vi "DB - Columns INFO.vi"(0 "Refnum in":T3, 1 "subVI (auto)":bool=TRUE, 5 "DB.dbo.Table":string="SRTRS.MasterData.Procedure", 11 "error in (no error)":errorcluster) -> (2 "IDENTITY COLUMN":string, 3 "Table Description":string, 4 "Refnum out":T3, 6 "COLUMN_NAME":string[](array[string]), 8 "DATA_TYPE":string[](array[string]), 10 "PRECISION":string[](array[string]), 13 "COUNT":i32, 14 "MS_Description":string[](array[string]), 15 "error out":errorcluster)   [LabVIEW 2013]
uses:
  <vilib>/addons/database/Connection.llb/Conn ObjectReference.ctl
  Controls/DB - DB.Schema.Table.ctl
  <vilib>/addons/database/Connection.llb/Conn Execute.vi
  <vilib>/addons/database/Recordset.llb/Rec Fetch String Data (R).vi
  <vilib>/addons/database/Recordset.llb/Rec Destroy - Connection.vi
  <vilib>/addons/database/Recordset.llb/Rec Fetch Recordset Data (R).vi
  <vilib>/addons/database/Connection.llb/DB Tools Open Connec (String).vi
  <vilib>/addons/database/_DB Variant To Data/Database Variant To Data.xnode
  <vilib>/addons/database/NI_Database_API.lvlib
panel:
  out "# of SQL Statements":i32
  out "Fetch = 0 Error":errorcluster
  out "isIdentity":string[](array[string])
  out "SQL Statement":string[](array[string])
  out "String":string
  out "DB.Schema.Table":T1
  out "call chain":string[](array[string])
  out "data":string[][](array[string])
  in  "Connection Information":T2={"Connection "="SQL Server 32bit HPEnvy", "Username"="admin", "Password"="admin123"}
  # "Orders\nPartsDetails\nTransactions"
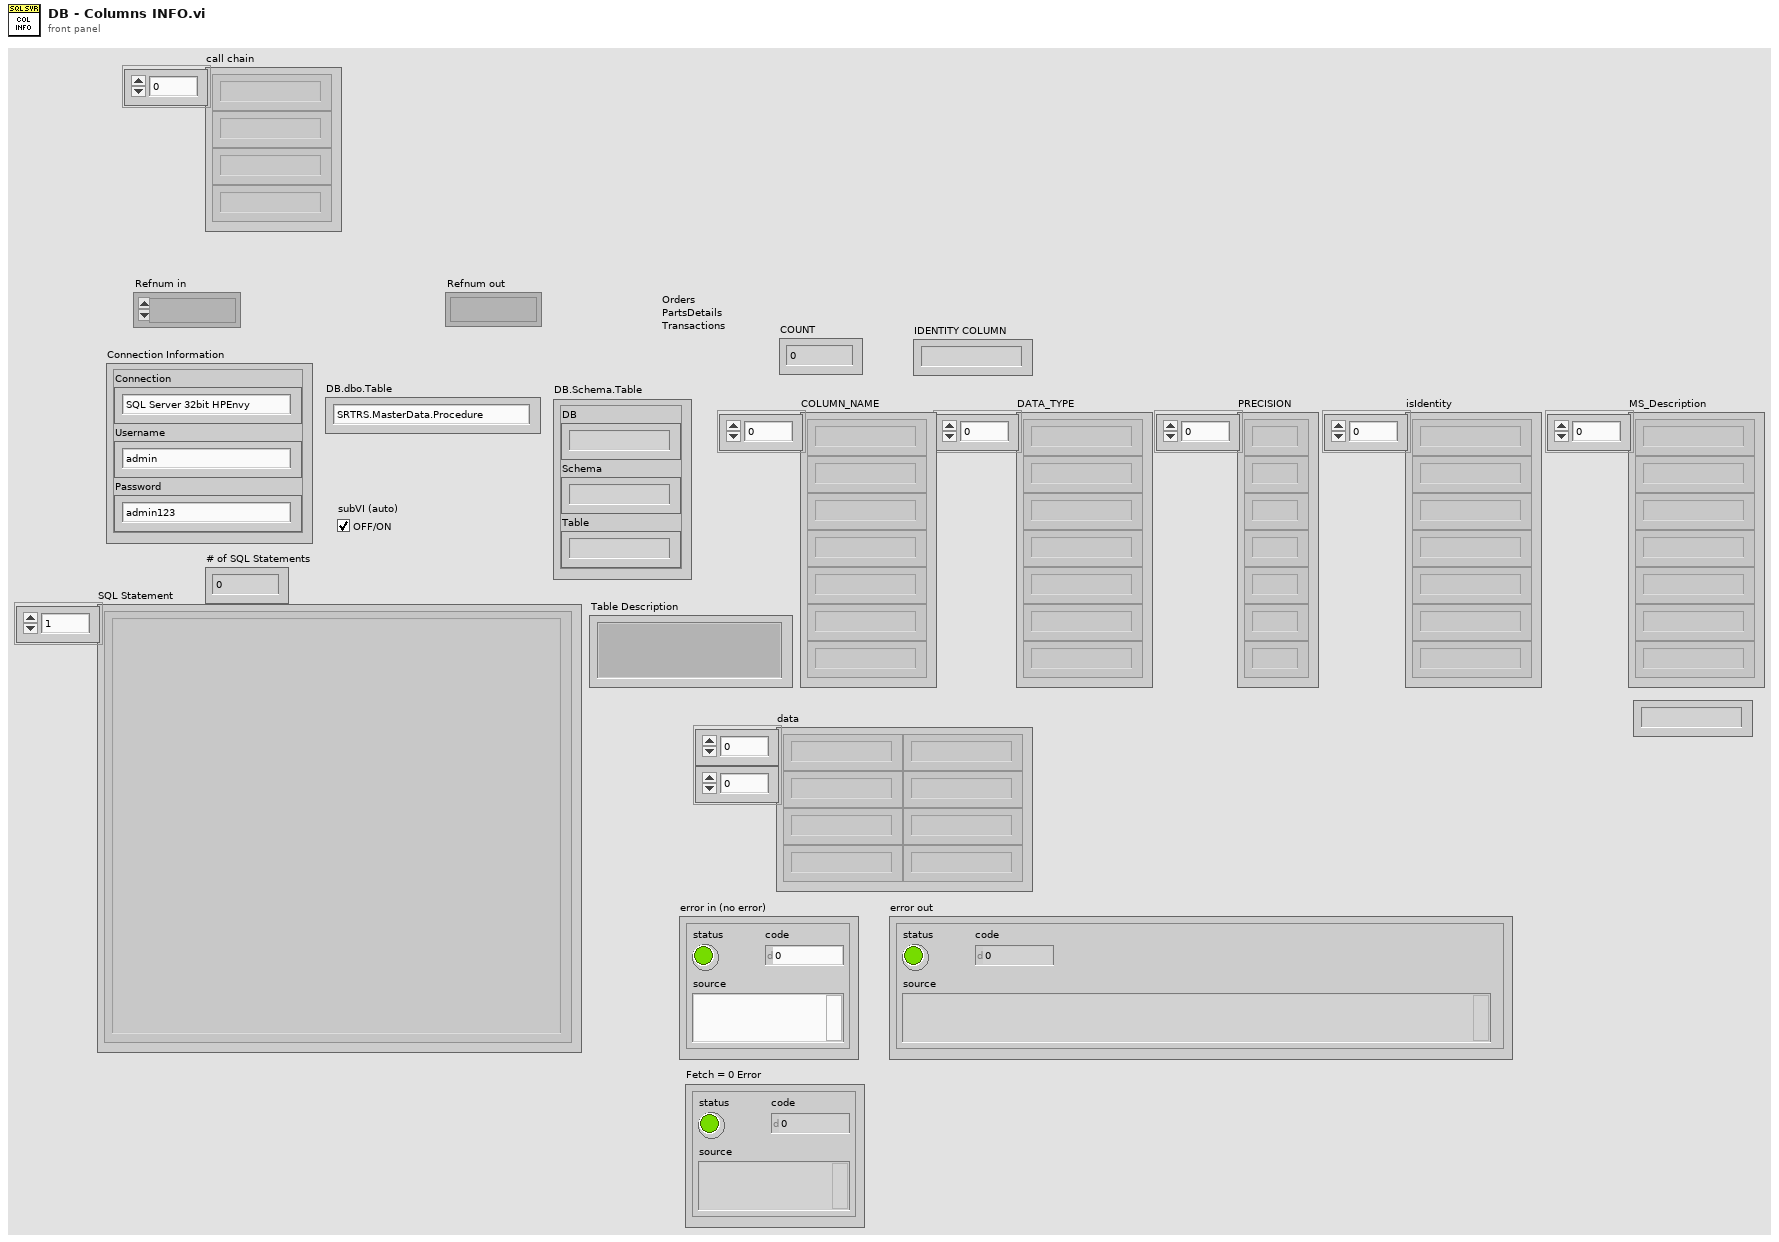
[diagram p1: front panel]
types:
  T1 = typedef "DB - DB.Schema.Table.ctl" = cluster{"DB":string, "Schema":string, "Table":string}
  T2 = cluster{"Connection ":string, "Username":string, "Password":string}
  T3 = typedef "NI_Database_API.lvlib/Conn ObjectReference.ctl" = refnum<k1>
  T4 = typedef "NI_Database_API.lvlib/Rec ObjectReference.ctl" = refnum<k1>
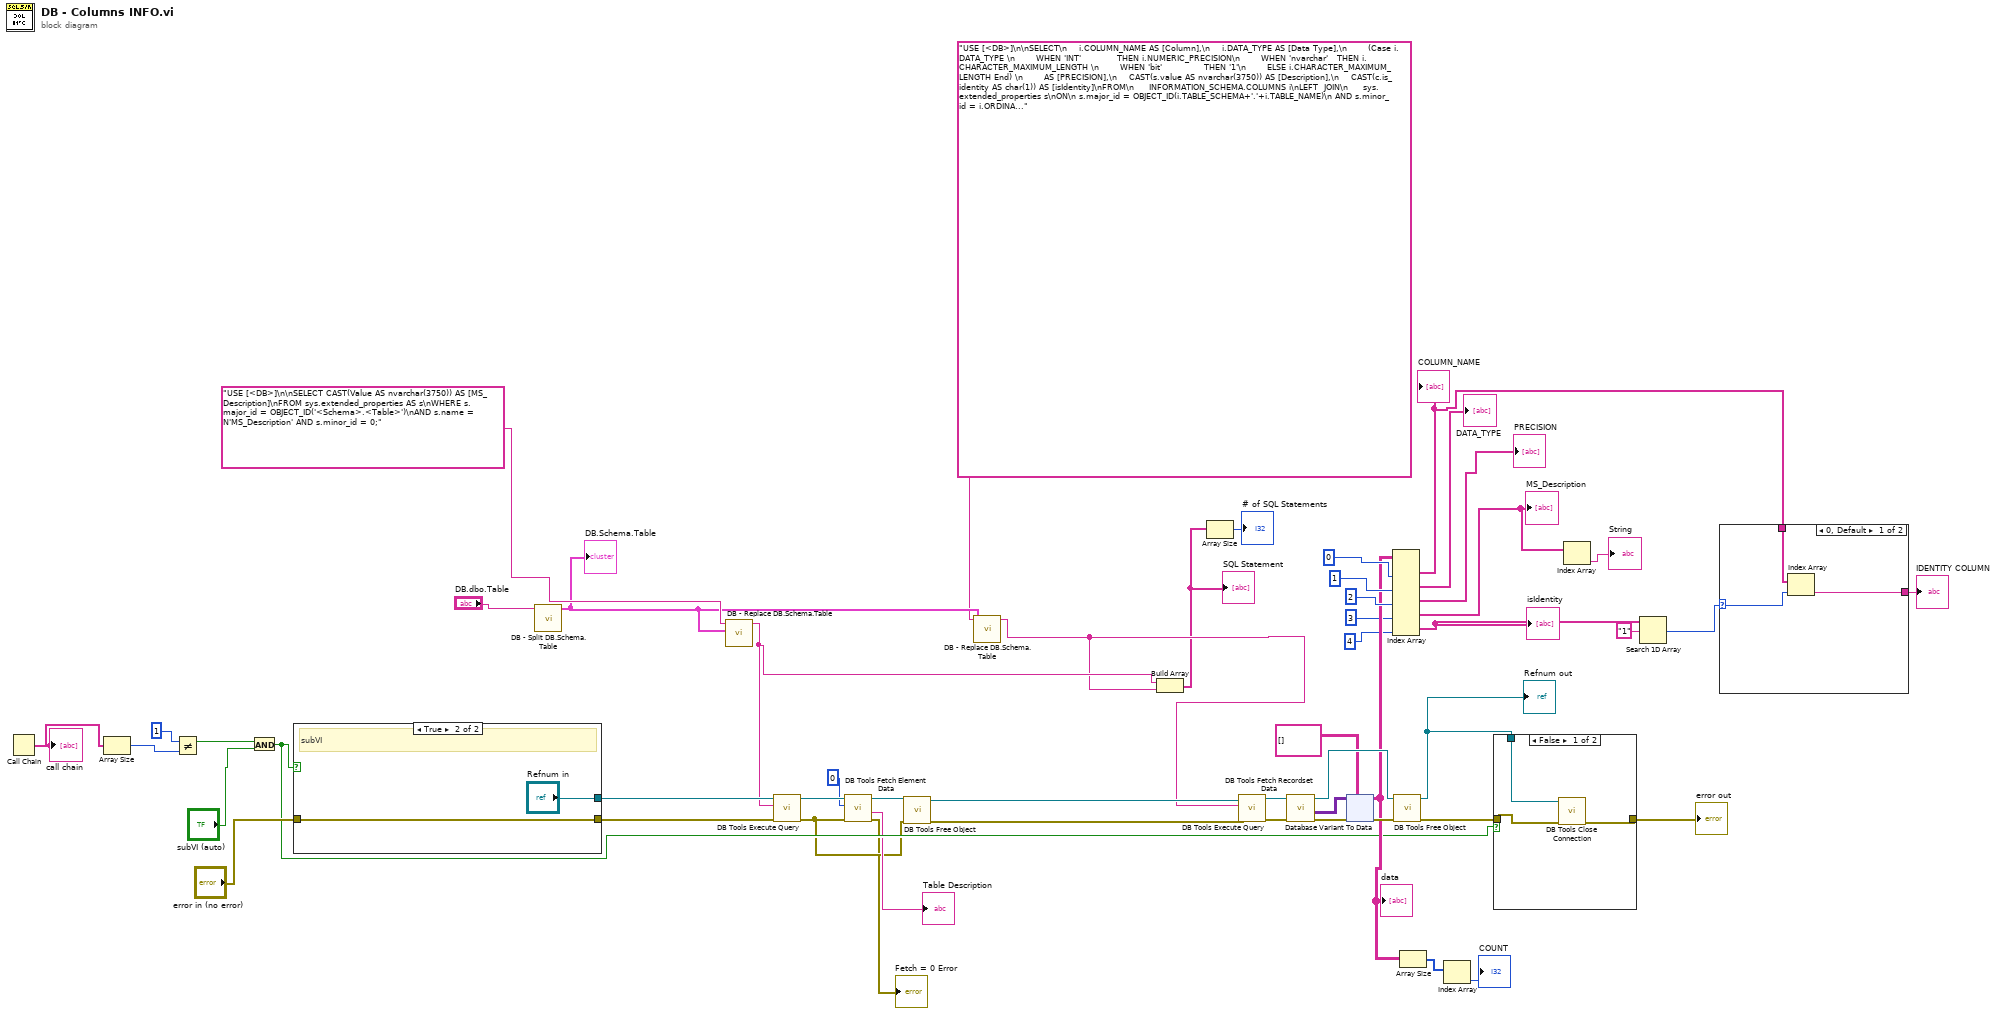
[diagram p0: block diagram]
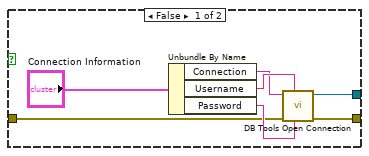
[diagram p4: hidden frame]
diagram:
  n1 = Call Chain() -> (call chain=w32:string[])
  "call chain" <- w32
  n2 = Array Size(array=w32) -> (size(s)=w31:i32)
  n3 = Not Equal?(x=1, y=w31) -> (x != y?=w30:bool)
  n4 = And(x=w30, y="subVI (auto)") -> (x .and. y?=w27:bool)
  n5 = case shown="True" w27 {
    tunnel: [w55 "Refnum in"] -> w21
    tunnel: "error in (no error)" -> [w54 w60]
    tunnel: [w53 w60] -> w20
    frame False {
      n6 = Unbundle By Name("Connection Information") -> ("Connection"=w57:string, "Username"=w58:string, "Password"=w56:string)
      n7 = call-poly <vilib>:"DB Tools Open Connection.vi"("password"=w56, "userID"=w58, "error in (no error)"=w54, "connection information"=w57) -> ("error out"=w53:errorcluster, "connection reference"=w55:T3)  [unwired: 4 in]
    }
    frame True {
      # "subVI"
    }
  }
  n8 = call "DB - Split DB.Schema.Table.vi"("DB.Schema.Table"="DB.dbo.Table") -> ("DB.Schema.Table"=w22:T1)  [unwired: 10 in]
  "DB.Schema.Table" <- w22
  n9 = call "DB - Replace DB.Schema.Table.vi"("DB.Schema.Table"=w22, "string in"="USE [<DB>]\n\nSELECT CAST(Value AS nvarchar(3750)) AS [MS_Description]\nFROM sys.extended_properties AS s\nWHERE s.major_id = OBJECT_ID('<Schema>.<Table>')\nAND s.name = N'MS_Description' AND s.minor_id = 0;") -> ("string out"=w16:string)  [unwired: 8 in, 1 out]
  n10 = call-poly <vilib>:"DB Tools Execute Query.vi"("error in (no error)"=w20, "SQL query"=w16, "connection reference"=w21) -> ("error out"=w4:errorcluster, "recordset reference"=w7:T4)  [unwired: 5 in]
  n11 = call-poly <vilib>:"DB Tools Fetch Element Data.vi"("error in (no error)"=w4, "column index"=0, "recordset reference"=w7) -> ("error out"=→"Fetch = 0 Error":errorcluster, "data"=→"Table Description":string, "recordset reference out"=w19:T4)  [unwired: 4 in]
  n12 = call-poly <vilib>:"DB Tools Free Object.vi"("error in (no error)"=w4, "recordset reference"=w19) -> ("error out"=w17:errorcluster, "connection reference"=w18:T3)  [unwired: 8 in]
  n13 = call "DB - Replace DB.Schema.Table.vi"("DB.Schema.Table"=w22, "string in"="USE [<DB>]\n\nSELECT\n    i.COLUMN_NAME AS [Column],\n    i.DATA_TYPE AS [Data Type],\n       (Case i.DATA_TYPE \n       WHEN 'INT'            THEN i.NUMERIC_PRECISION\n       WHEN 'nvarchar'   THEN i.CHARACTER_MAXIMUM_LENGTH \n       WHEN 'bit'              THEN '1'\n       ELSE i.CHARACTER_MAXIMUM_LENGTH End) \n       AS [PRECISION],\n    CAST(s.value AS nvarchar(3750)) AS [Description],\n    CAST(c.is_identity AS char(1)) AS [isIdentity]\nFROM\n     INFORMATION_SCHEMA.COLUMNS i\nLEFT  JOIN\n     sys.extended_properties s\nON\n s.major_id = OBJECT_ID(i.TABLE_SCHEMA+'.'+i.TABLE_NAME)\n AND s.minor_id = i.ORDINAL_POSITION\n AND s.name = 'MS_Description'\n\nJOIN sys.columns c\nON\ni.COLUMN_NAME= c.name AND\nOBJECT_ID(i.TABLE_SCHEMA+'.'+i.TABLE_NAME) = c.object_id\n\nWHERE\n i.TABLE_SCHEMA = '<Schema>' AND   i.TABLE_NAME = '<Table>'\nORDER BY\n i.TABLE_NAME, i.ORDINAL_POSITION\n" ("string")) -> ("string out"=w15:string)  [unwired: 8 in, 1 out]
  n14 = Build Array(w16, w15) -> (w2:string[])
  "SQL Statement" <- w2
  n15 = Array Size(array=w2) -> (size(s)=→"# of SQL Statements":i32)
  n16 = call-poly <vilib>:"DB Tools Execute Query.vi"("error in (no error)"=w17, "SQL query"=w15, "connection reference"=w18) -> ("error out"=w49:errorcluster, "recordset reference"=w47:T4)  [unwired: 5 in]
  n17 = call-poly <vilib>:"DB Tools Fetch Recordset Data.vi"("error in (no error)"=w49, "recordset reference"=w47) -> ("error out"=w51:errorcluster, "recordset data"=w50:variant[][], "recordset reference out"=w48:T4)  [unwired: 3 in]
  n18 = xnode "Database Variant To Data"("database variant"=w50, "error in (no error)"=w51, "type"=string[][] []) -> ("data"=w35:string[][], "error out"=w52:errorcluster)
  "data" <- w35
  n19 = Index Array(array=w35, index (col) #1=0 ("index (row)"), index (col) #2=1 ("disabled index (row)"), index (col) #3=2 ("index (col)"), index (col) #4=3 ("index (col)"), index (col) #5=4 ("index (col)")) -> (element #1=w9:string[], element #2=→"DATA_TYPE":string[], element #3=→"PRECISION":string[], element #4=w25:string[], element #5=w12:string[])  [unwired: 5 in]
  "COLUMN_NAME" <- w9
  "MS_Description" <- w25
  "isIdentity" <- w12
  n20 = call-poly <vilib>:"DB Tools Free Object.vi"("error in (no error)"=w52, "recordset reference"=w48) -> ("error out"=w44:errorcluster, "connection reference"=w42:T3)  [unwired: 8 in]
  "Refnum out" <- w42
  n21 = Array Size(array=w35) -> (size(s)=w34:i32[])
  n22 = Index Array(array=w34) -> (element=→"COUNT":i32)  [unwired: 1 in]
  n23 = case shown="False" w27 {
    tunnel: w42 -> [w64 _]
    tunnel: w44 -> [w63 w65]
    tunnel: [w62 w65] -> w45
    frame False {
      n24 = call <vilib>:"DB Tools Close Connection.vi"("error in (no error)"=w63, "connection reference"=w64) -> ("error out"=w62:errorcluster)  [unwired: 5 in]
    }
    frame True {
      # "subVI"
    }
  }
  "error out" <- w45
  n25 = Index Array(array=w25) -> (element=→"String":string)  [unwired: 1 in]
  n26 = Search 1D Array(1D array=w12, element="1") -> (index of element=w10:i32)  [unwired: 1 in]
  n27 = case shown="0, Default" w10 {
    selector: w10 -> [w67 _]
    tunnel: w9 -> [w68 _]
    tunnel: [w66 _] -> w8
    frame 0, Default {
      n28 = Index Array(array=w68, index=w67) -> (element=w66:string)
    }
    frame -1 {
    }
  }
  "IDENTITY COLUMN" <- w8
